vi "Laser Power Ctrl Wavelength to Notifier Name.vi"(7 "Wavelength":u16) -> (8 "Notifier Name":string, 15 "Wavelength":string)   [LabVIEW 2016]
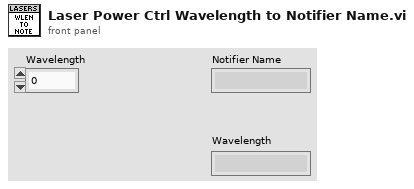
[diagram p1: front panel]
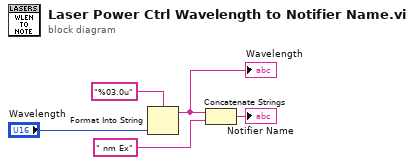
[diagram p0: block diagram]
diagram:
  n1 = Format Into String(format string="%03.0u", "Wavelength") -> (resulting string=w1:string)  [unwired: 2 in, 1 out]
  "Wavelength" <- w1
  n2 = Concatenate Strings(w1, " nm Ex") -> (→"Notifier Name":string)
